vi "Snare_Ram.vi"(10 "M":fxp<+,32,32>, 11 "Trigger":bool) -> (3 "Ram Out":fxp<+/-,8,8>)   [LabVIEW 2015]
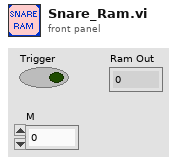
[diagram p1: front panel]
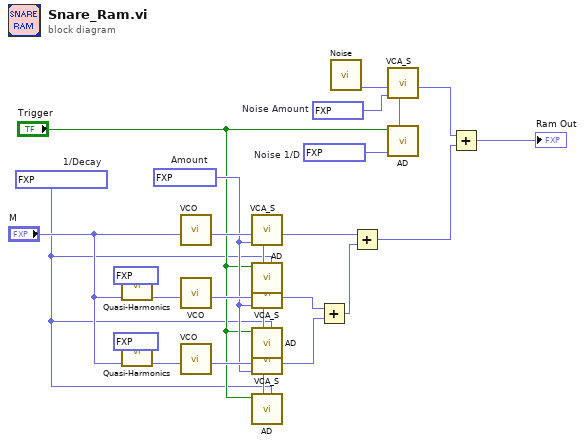
[diagram p0: block diagram]
diagram:
  w9 = fxp<+,8,0> 0.89453125  # Noise Amount
  w7 = fxp<+,16,0> 4.57763671875e-05  # Noise 1/D
  w8 = fxp<+,8,0> 0.99609375  # Amount
  w1 = fxp<+,16,0> 3.0517578125e-05  # 1/Decay
  n1 = call "Quasi-Harmonics.vi"("Relative Freq"=fxp<+,8,3> 1.09375 ("relative f"), "1st partial"="M") -> ("Result Partial"=w21:fxp<+,32,32>)  [unwired: 9 in]
  n2 = call "Quasi-Harmonics.vi"("Relative Freq"=fxp<+,8,3> 1.21875 ("relative f"), "1st partial"="M") -> ("Result Partial"=w22:fxp<+,32,32>)  [unwired: 9 in]
  n3 = call "VCO.vi"("M"="M") -> ("Sine Sample"=w11:fxp<+/-,8,8>)  [unwired: 10 in]
  n4 = call "VCO.vi"("M"=w21) -> ("Sine Sample"=w10:fxp<+/-,8,8>)  [unwired: 10 in]
  n5 = call "VCO.vi"("M"=w22) -> ("Sine Sample"=w12:fxp<+/-,8,8>)  [unwired: 10 in]
  n6 = call "AD.vi"("1/Decay"=w1, "Trigger"="Trigger") -> ("Sample Out"=w5:fxp<+,8,0>)  [unwired: 9 in]
  n7 = call "VCA_S.vi"("EG"=w5, "Amount"=w8, "Sample In"=w11) -> ("Sample Out"=w18:fxp<+/-,8,8>)  [unwired: 8 in]
  n8 = call "AD.vi"("1/Decay"=w1, "Trigger"="Trigger") -> ("Sample Out"=w2:fxp<+,8,0>)  [unwired: 9 in]
  n9 = call "VCA_S.vi"("EG"=w2, "Amount"=w8, "Sample In"=w10) -> ("Sample Out"=w14:fxp<+/-,8,8>)  [unwired: 8 in]
  n10 = call "AD.vi"("1/Decay"=w1, "Trigger"="Trigger") -> ("Sample Out"=w3:fxp<+,8,0>)  [unwired: 9 in]
  n11 = call "VCA_S.vi"("EG"=w3, "Amount"=w8, "Sample In"=w12) -> ("Sample Out"=w13:fxp<+/-,8,8>)  [unwired: 8 in]
  n12 = Add(x=w14, y=w13) -> (x+y=w15:fxp<+/-,8,8>)
  n13 = call "Noise.vi"() -> ("White Noise Out"=w16:fxp<+/-,8,8>)  [unwired: 11 in]
  n14 = Add(x=w18, y=w15) -> (x+y=w19:fxp<+/-,8,8>)
  n15 = call "AD.vi"("1/Decay"=w7, "Trigger"="Trigger") -> ("Sample Out"=w6:fxp<+,8,0>)  [unwired: 9 in]
  n16 = call "VCA_S.vi"("EG"=w6, "Amount"=w9, "Sample In"=w16) -> ("Sample Out"=w17:fxp<+/-,8,8>)  [unwired: 8 in]
  n17 = Add(x=w17, y=w19) -> (x+y=→"Ram Out":fxp<+/-,8,8>)
